vi "test FGV_SubPannel.vi"() -> ()   [LabVIEW 2017]
uses:
  FGV_SubPannel/Func_Subpannel.ctl
panel:
  in  "stop":bool
  in  "VI to Display":u16(ring) items=["Sine Graph", "Random Data Chart", "Current Time"]
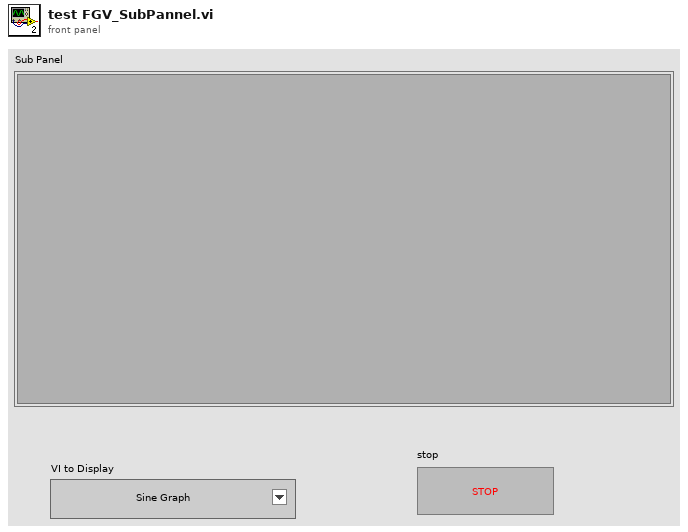
[diagram p1: front panel]
types:
  T1 = typedef "Func_Subpannel.ctl" = enum16{"Initialize", "Get all Opend VIs", "Update Insert VI", "Close all VIs"}
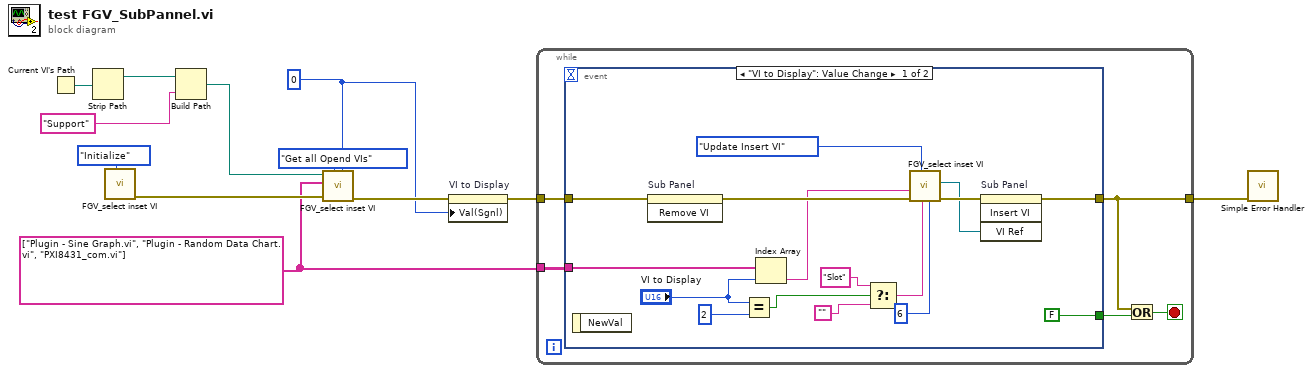
[diagram p0: block diagram]
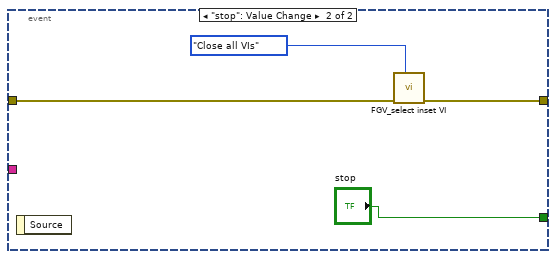
[diagram p2: hidden frame]
diagram:
  w8 = 0
  w6 = string[] ["Plugin - Sine Graph.vi", "Plugin - Random Data Chart.vi", "PXI8431_com.vi"]
  n1 = Current VI's Path() -> (path=w4:path)
  n2 = Strip Path(path=w4) -> (stripped path=w3:path)  [unwired: 1 out]
  n3 = call "FGV_select inset VI.vi"("Function"=Func_Subpannel."Initialize") -> ("error out"=w11:errorcluster)  [unwired: 9 in, 1 out]
  n4 = Build Path(base path=w3, name or relative path="Support") -> (appended path=w1:path)
  n5 = call "FGV_select inset VI.vi"("First Run"=w8, "Function"=Func_Subpannel."Get all Opend VIs", "error in (no error)"=w11, "VIs Name"=w6, "ModulesPath"=w1) -> ("error out"=w9:errorcluster)  [unwired: 5 in, 1 out]
  n6 = property on="VI to Display" class="Ring (strict)"(error in=w9, "Val(Sgnl)"=w8) -> (error out=w7:errorcluster)  [unwired: 1 in, 1 out]
  n7 = while {
    tunnel: w7 -> [w17]
    tunnel: w6 -> [w16]
    tunnel: [w15] -> w5
    stop <- w14 stop-if-true
    n8 = event shown="[0] \"VI to Display\": Value Change" {
      selector: _ -> [_ _]
      dyn-events: _ -> [_ _]
      timeout: _ -> [_ _]
      tunnel: w17 -> [w33 w36]
      tunnel: w16 -> [w30 _]
      tunnel: [w26 w35] -> w15
      tunnel: [FALSE "stop"] -> w13
      event "VI to Display": Value Change {
        n9 = event-data() -> ()  [unwired: 1 in, 1 out]
        n10 = invoke on="Sub Panel" class="SubPnl" method="Remove VI"(error in=w33) -> (error out=w32:errorcluster)  [unwired: 2 in, 2 out]
        n11 = Equal?(x="VI to Display", y=2) -> (x = y?=w22:bool)
        n12 = Index Array(array=w30, index="VI to Display") -> (element=w29:string)
        n13 = Select(t="Slot", s=w22, f="") -> (s? t:f=w19:string)
        n14 = call "FGV_select inset VI.vi"("Value"=6, "Parameter"=w19, "Function"=Func_Subpannel."Update Insert VI", "error in (no error)"=w32, "Inser VI name"=w29) -> ("error out"=w28:errorcluster, "Inset VI"=w27:refnum<vi>)  [unwired: 5 in]
        n15 = invoke on="Sub Panel" class="SubPnl" method="Insert VI"(error in=w28, "VI Ref"=w27) -> (error out=w26:errorcluster)  [unwired: 2 in, 3 out]
      }
      event "stop": Value Change {
        n16 = event-data() -> ()  [unwired: 1 in, 1 out]
        n17 = call "FGV_select inset VI.vi"("Function"=Func_Subpannel."Close all VIs", "error in (no error)"=w36) -> ("error out"=w35:errorcluster)  [unwired: 8 in, 1 out]
      }
    }
    n18 = Or(x=w15, y=w13) -> (x .or. y?=w14:bool)
  }
  n19 = call <vilib>:"Simple Error Handler.vi"("error in (no error)"=w5) -> ()  [unwired: 4 in, 5 out]
